vi "Init Picture.vi"(8 "error in (no error)":errorcluster, 9 "New Object":refnum<class "Graphics Object.lvclass">, 10 "Previous Picture":refnum<class "Picture.lvclass">, 11 "Picture in":refnum<class "Picture.lvclass">) -> (0 "error out":errorcluster, 3 "Picture out":refnum<class "Picture.lvclass">)   [LabVIEW 2018, in "Picture.lvclass"]
doc: "Initialize a picture"
uses:
  Picture.lvclass
  Graphics Object/Graphics Object.lvclass
  Picture.lvclass/Picture.ctl
panel:
  # "expressionflow.com"
  # "Copyright (c) 2008 Tomi Maila. All rights reserved."
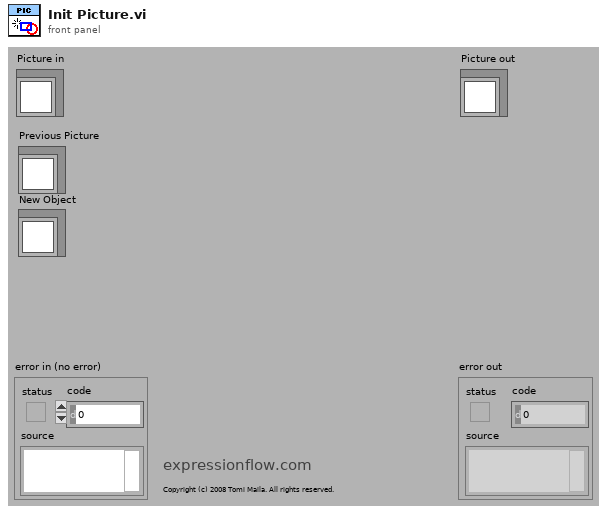
[diagram p1: front panel]
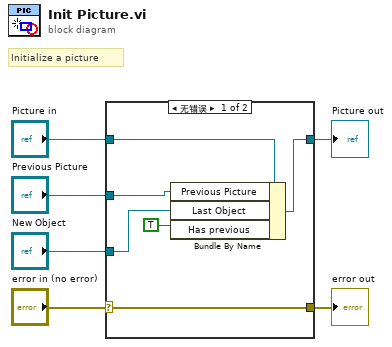
[diagram p0: block diagram]
diagram:
  # "Initialize a picture"
  n1 = case shown="无错误" "error in (no error)" {
    selector: "error in (no error)" -> [w12 w14]
    tunnel: [w12 w14] -> w5
    tunnel: [w10 w13] -> w3
    tunnel: "Picture in" -> [w11 w13]
    tunnel: "Previous Picture" -> [w9 _]
    tunnel: "New Object" -> [w8 _]
    frame No Error {
      n2 = Bundle By Name(cluster=w11, "Previous Picture"=w9, "Last Object"=w8, "Has previous"=TRUE) -> (w10:refnum<class "Picture.lvclass">)
    }
    frame Error {
    }
  }
  "error out" <- w5
  "Picture out" <- w3
